vi "Get Plugin Paths.vi"(8 "error in":errorcluster, 11 "measurement in":refnum<class "Continuous Counting Measurement2.lvclass">) -> (0 "error out":errorcluster, 2 "plugin paths":T1, 3 "measurement out":refnum<class "Continuous Counting Measurement2.lvclass">)   [LabVIEW 2021, in "MeasurementServerTests.lvlib" / "Measurement Service Tests.lvlib" / "Continuous Counting Measurement2.lvclass"]
uses:
  Continuous Counting Measurement2.lvclass
  Continuous Counting Measurement2.lvclass/Continuous Counting Measurement2.ctl
  Runtime/Measurements/Measurement Plugin Service/Plugin Paths.ctl
  Runtime/Measurements/Measurement Plugin Service/Measurement Plugin Service.lvclass
  Measurement Logic.vi
  Measurement Configuration.ctl
  Measurement Results.ctl
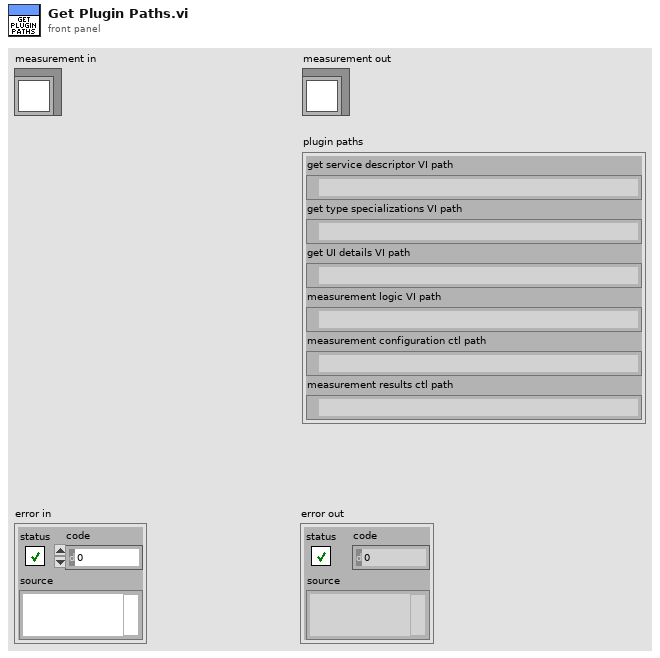
[diagram p1: front panel]
types:
  T1 = typedef "NI Measurement Plug-In SDK.lvlib/Measurement Plugin Service.lvclass/Plugin Paths.ctl" = cluster{"get service descriptor VI path":path, "get type specializations VI path":path, "get UI details VI path":path, "measurement logic VI path":path, "measurement configuration ctl path":path, "measurement results ctl path":path}
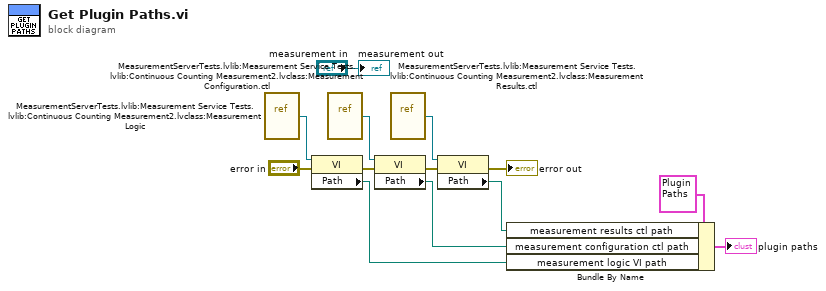
[diagram p0: block diagram]
diagram:
  n1 = vi-ref "MeasurementServerTests.lvlib:Measurement Service Tests.lvlib:Continuous Counting Measurement2.lvclass:Measurement Logic.vi"() -> (w9:refnum<vi>)
  n2 = property class="VI"(reference=w9, error in="error in") -> (error out=w1:errorcluster, "Path"=w6:path)  [unwired: 1 out]
  n3 = vi-ref "MeasurementServerTests.lvlib:Measurement Service Tests.lvlib:Continuous Counting Measurement2.lvclass:Measurement Configuration.ctl"() -> (w7:refnum<vi>)
  n4 = property class="VI"(reference=w7, error in=w1) -> (error out=w13:errorcluster, "Path"=w12:path)  [unwired: 1 out]
  n5 = vi-ref "MeasurementServerTests.lvlib:Measurement Service Tests.lvlib:Continuous Counting Measurement2.lvclass:Measurement Results.ctl"() -> (w8:refnum<vi>)
  n6 = property class="VI"(reference=w8, error in=w13) -> (error out=→"error out":errorcluster, "Path"=w11:path)  [unwired: 1 out]
  n7 = Bundle By Name(cluster=T1 {"get service descriptor VI path"=path "", "get type specializations VI path"=path "", "get UI details VI path"=path "", "measurement logic VI path"=path "", "measurement configuration ctl path"=path "", "measurement results ctl path"=path ""} ("plugin paths"), "measurement results ctl path"=w11, "measurement configuration ctl path"=w12, "measurement logic VI path"=w6) -> (→"plugin paths":T1)
  "measurement out" <- "measurement in"
